vi "Save 6-Contact Sample test results to Disk.vi"(0 "Save To Path":path, 1 "Sample Name":string, 2 "User Name":string, 3 "Test Date":string, 5 "Test Settings":T4={"Current Level"=0.0, "Compliance Level"=0.0, "Soak Time"=0.0, "NPLC Voltmeter"=1.0, "Count Voltmeter"=1, "NPLC Ammeter"=1.0, "Count Ammeter"=1, "Sample Resistivity"=enum."Low", "Sample Thickness"=0.0, "Magnetic Flux"=0.0, "Units"=enum."T", "Sample Dimensions x"=0.0, "Sample Dimensions y"=0.0, "Sample Dimensions D1"=0.0, "Sample Dimensions D2"=0.0, "Sample Width Ws"=0.0, "Slot Number of 3765 card"=1} {"Slot Number of 3765 card" min=1 max=6; "NPLC Ammeter" min=0.01 max=10.0; "NPLC Voltmeter" min=0.01 max=10.0 format="%^#_6g"; "Count Ammeter" min=1 max=1024; "Count Voltmeter" min=1 max=1024; "Soak Time" format="%^#_6g"; "Compliance Level" format="%^#_6g"; "Current Level" format="%^#_6e"}, 11 "error in (no error)":errorcluster, 12 "6-Contact Sample Resitivity Measurements":cluster{"V1":dbl, "V2":dbl, "V3":dbl, "V4":dbl}, 13 "6-Contact Sample Hall Voltage Measurements":T2, 14 "6-Contact Sample Results":T1) -> (15 "error out":errorcluster)   [LabVIEW 2016]
uses:
  Hall Effect Library/Public/Controls/Resisitivity.ctl
  Hall Effect Library/Hall Effect Library.lvlib
panel:
  # "Resistivity"
  # "Hall Coefficient"
  # "Hall Mobility"
  # "Ohm cm"
  # "RAvg"
  # "PAvg"
  # "cm^3/C"
  # "uH"
  # "cm^2/V s"
  # "Ohm cm"
  # "PA"
  # "RH1"
  # "cm^3/C"
  # "PB"
  # "RH2"
  # "Ohm cm"
  # "cm^3/C"
  # "Magnet"
  # "V1"
  # "V2"
  # "V3"
  # "V4"
  # "Pos"
  # "Neg"
  # "Polarity"
  # "V5"
  # "V6"
  # "V7"
  # "V8"
  # "V1"
  # "Currents"
  # "V2"
  # "Pos"
  # "Volts"
  # "Neg"
  # "Direction"
  # "V4"
  # "V3"
  # "NPLC"
  # "A"
  # "V"
  # "s"
  # "Measure Count"
  # "cm"
  # "cm"
  # "cm"
  # "cm"
  # "cm"
  # "cm"
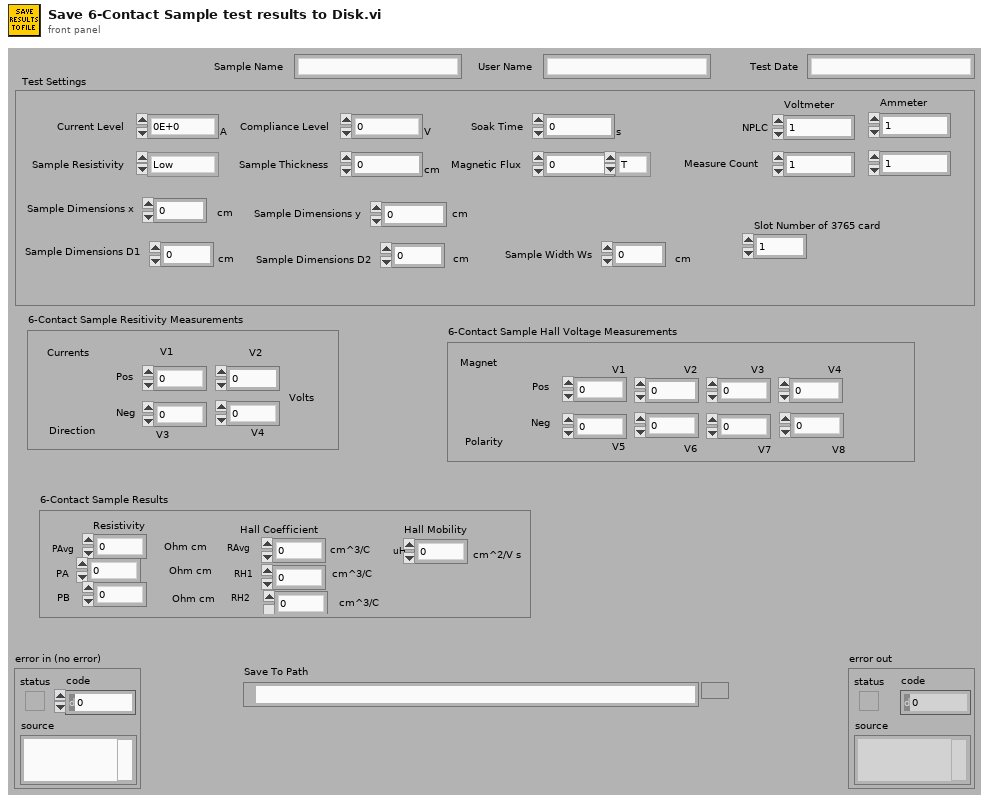
[diagram p1: front panel]
types:
  T1 = cluster{"Pavg":dbl, "PA":dbl, "PB":dbl, "RAVG":dbl, "RH1":dbl, "RH2":dbl, "uH":dbl}
  T2 = cluster{"V1":dbl, "V2":dbl, "V3":dbl, "V4":dbl, "V5":dbl, "V6":dbl, "V7":dbl, "V8":dbl}
  T3 = typedef "Hall Effect Library.lvlib/Resisitivity.ctl" = enum16{"Low", "High"}
  T4 = cluster{"Current Level":dbl, "Compliance Level":dbl, "Soak Time":dbl, "NPLC Voltmeter":dbl, "Count Voltmeter":i32, "NPLC Ammeter":dbl, "Count Ammeter":i32, "Sample Resistivity":T3, "Sample Thickness":dbl, "Magnetic Flux":dbl, "Units":enum16{"Gs", "T"}, "Sample Dimensions x":dbl, "Sample Dimensions y":dbl, "Sample Dimensions D1":dbl, "Sample Dimensions D2":dbl, "Sample Width Ws":dbl, "Slot Number of 3765 card":u16}
  T5 = enum16{"open", "replace", "create", "open or create", "replace or create", "replace or create with confirmation"}
  T6 = cluster{"6-Contact Sample Resistivity Currents[0]":dbl, "6-Contact Sample Resistivity Currents[1]":dbl, "6-Contact Sample Resistivity Currents[2]":dbl, "6-Contact Sample Resistivity Currents[3]":dbl}
  T7 = cluster{"6-Contact Sample Hall Currents[0]":dbl, "6-Contact Sample Hall Currents[1]":dbl, "6-Contact Sample Hall Currents[2]":dbl, "6-Contact Sample Hall Currents[3]":dbl, "6-Contact Sample Hall Currents[4]":dbl, "6-Contact Sample Hall Currents[5]":dbl, "6-Contact Sample Hall Currents[6]":dbl, "6-Contact Sample Hall Currents[7]":dbl}
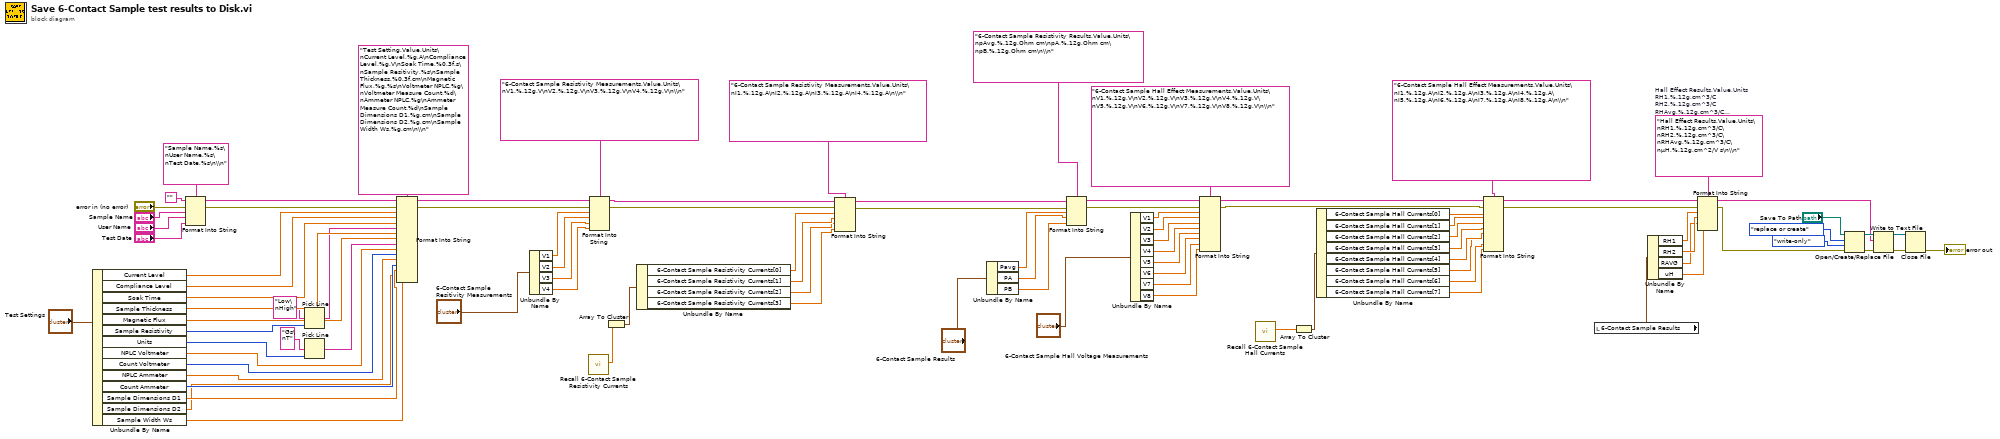
[diagram p0: block diagram]
diagram:
  w60 = "Hall Effect Results,Value,Units\nRH1,%.12g,cm^3/C\nRH2,%.12g,cm^3/C\nRHAvg,%.12g,cm^3/C\nµH,%.12g,cm^2/V s\n\\n"  # Hall Effect Results,Value,Units RH1,%.12g,cm^3/C RH2,%.12g,cm^3/C RHAvg,%.12g,cm^3/C µH,%.12g,cm^2/V s \n
  n1 = Unbundle By Name("Test Settings") -> ("Current Level"=w88:dbl, "Compliance Level"=w87:dbl, "Soak Time"=w86:dbl, "Sample Thickness"=w85:dbl, "Magnetic Flux"=w84:dbl, "Sample Resistivity"=w80:T3, "Units"=w81:enum16{"Gs", "T"}, "NPLC Voltmeter"=w48:dbl, "Count Voltmeter"=w47:i32, "NPLC Ammeter"=w46:dbl, "Count Ammeter"=w45:i32, "Sample Dimensions D1"=w44:dbl, "Sample Dimensions D2"=w43:dbl, "Sample Width Ws"=w42:dbl)
  n2 = Format Into String(format string="Sample Name,%s\nUser Name,%s\nTest Date,%s\n\\n", initial string="", error in="error in (no error)", "Sample Name", "User Name", "Test Date") -> (resulting string=w76:string, error out=w77:errorcluster)
  n3 = Pick Line(multi-line string="Low\nHigh", line index=w80) -> (output string=w79:string)  [unwired: 1 out]
  n4 = Pick Line(multi-line string="Gs\nT", line index=w81) -> (output string=w78:string)  [unwired: 1 out]
  n5 = Format Into String(format string="Test Setting,Value,Units\nCurrent Level,%g,A\nCompliance Level,%g,V\nSoak Time,%0.3f,s\nSample Resitivity,%s\nSample Thickness,%0.3f,cm\nMagnetic Flux,%g,%s\nVoltmeter NPLC,%g\nVoltmeter Measure Count,%d\nAmmeter NPLC,%g\nAmmeter Measure Count,%d\nSample Dimensions D1,%g,cm\nSample Dimensions D2,%g,cm\nSample Width Ws,%g,cm\n\\n", initial string=w76, error in=w77, w88, w87, w86, w79, w85, w84, w78, w48, w47, w46, w45, w44, w43, w42) -> (resulting string=w74:string, error out=w73:errorcluster)
  n6 = Unbundle By Name("6-Contact Sample Resitivity Measurements") -> ("V1"=w40:dbl, "V2"=w39:dbl, "V3"=w38:dbl, "V4"=w37:dbl)
  n7 = call "Recall 6-Contact Sample Resistivity Currents.vi"() -> ("6-Contact Sample Resistivity Currents"=w26:dbl[])  [unwired: 11 in]
  n8 = Format Into String(format string="6-Contact Sample Resistivity Measurements,Value,Units\nV1,%.12g,V\nV2,%.12g,V\nV3,%.12g,V\nV4,%.12g,V\n\\n", initial string=w74, error in=w73, w40, w39, w38, w37) -> (resulting string=w20:string, error out=w19:errorcluster)
  n9 = Array To Cluster(array=w26) -> (cluster=w25:T6)
  n10 = Unbundle By Name(w25) -> ("6-Contact Sample Resistivity Currents[0]"=w24:dbl, "6-Contact Sample Resistivity Currents[1]"=w23:dbl, "6-Contact Sample Resistivity Currents[2]"=w22:dbl, "6-Contact Sample Resistivity Currents[3]"=w21:dbl)
  n11 = Format Into String(format string="6-Contact Sample Resistivity Measurements,Value,Units\nI1,%.12g,A\nI2,%.12g,A\nI3,%.12g,A\nI4,%.12g,A\n\\n", initial string=w20, error in=w19, w24, w23, w22, w21) -> (resulting string=w18:string, error out=w17:errorcluster)
  n12 = Unbundle By Name("6-Contact Sample Results") -> ("Pavg"=w35:dbl, "PA"=w34:dbl, "PB"=w33:dbl)
  n13 = Format Into String(format string="6-Contact Sample Resistivity Results,Value,Units\npAvg,%.12g,Ohm cm\npA,%.12g,Ohm cm\npB,%.12g,Ohm cm\n\\n", initial string=w18, error in=w17, w35, w34, w33) -> (resulting string=w62:string, error out=w61:errorcluster)
  n14 = Unbundle By Name("6-Contact Sample Hall Voltage Measurements") -> ("V1"=w65:dbl, "V2"=w66:dbl, "V3"=w67:dbl, "V4"=w68:dbl, "V5"=w69:dbl, "V6"=w70:dbl, "V7"=w71:dbl, "V8"=w72:dbl)
  n15 = Format Into String(format string="6-Contact Sample Hall Effect Measurements,Value,Units\nV1,%.12g,V\nV2,%.12g,V\nV3,%.12g,V\nV4,%.12g,V\nV5,%.12g,V\nV6,%.12g,V\nV7,%.12g,V\nV8,%.12g,V\n\\n", initial string=w62, error in=w61, w65, w66, w67, w68, w69, w70, w71, w72) -> (resulting string=w5:string, error out=w4:errorcluster)
  n16 = call "Recall 6-Contact Sample Hall Currents.vi"() -> ("6-Contact Sample Hall Currents"=w15:dbl[])  [unwired: 11 in]
  n17 = Array To Cluster(array=w15) -> (cluster=w14:T7)
  n18 = Unbundle By Name(w14) -> ("6-Contact Sample Hall Currents[0]"=w13:dbl, "6-Contact Sample Hall Currents[1]"=w12:dbl, "6-Contact Sample Hall Currents[2]"=w11:dbl, "6-Contact Sample Hall Currents[3]"=w10:dbl, "6-Contact Sample Hall Currents[4]"=w9:dbl, "6-Contact Sample Hall Currents[5]"=w8:dbl, "6-Contact Sample Hall Currents[6]"=w7:dbl, "6-Contact Sample Hall Currents[7]"=w6:dbl)
  n19 = Format Into String(format string="6-Contact Sample Hall Effect Measurements,Value,Units\nI1,%.12g,A\nI2,%.12g,A\nI3,%.12g,A\nI4,%.12g,A\nI5,%.12g,A\nI6,%.12g,A\nI7,%.12g,A\nI8,%.12g,A\n\\n", initial string=w5, error in=w4, w13, w12, w11, w10, w9, w8, w7, w6) -> (resulting string=w3:string, error out=w2:errorcluster)
  n20 = local read "6-Contact Sample Results"() -> (w31:T1)
  n21 = Unbundle By Name(w31) -> ("RH1"=w30:dbl, "RH2"=w29:dbl, "RAVG"=w28:dbl, "uH"=w27:dbl)
  n22 = Format Into String(format string=w60, initial string=w3, error in=w2, w30, w29, w28, w27) -> (resulting string=w51:string, error out=w52:errorcluster)
  n23 = Open/Create/Replace File(file path (use dialog)="Save To Path", error in=w52, operation (0:open)=T5."replace or create", access (0:read/write)=enum16{"read/write", "read-only", "write-only"}."write-only") -> (refnum out=w56:refnum<file>, error out=w55:errorcluster)  [unwired: 3 out]
  n24 = Write to Text File(file (use dialog)=w56, text=w51, error in=w55) -> (refnum out=w53:refnum<file>, error out=w54:errorcluster)  [unwired: 2 out]
  n25 = Close File(refnum=w53, error in=w54) -> (error out=→"error out":errorcluster)  [unwired: 1 out]
